vi "Untitled 1.vi"() -> ()   [LabVIEW 2015]
uses:
  <vilib>/Utility/file.llb/Read Delimited Spreadsheet (DBL).vi
panel:
  out "Multiple Plots (custom time base)":dbl[](graph)
  in  "stop":bool
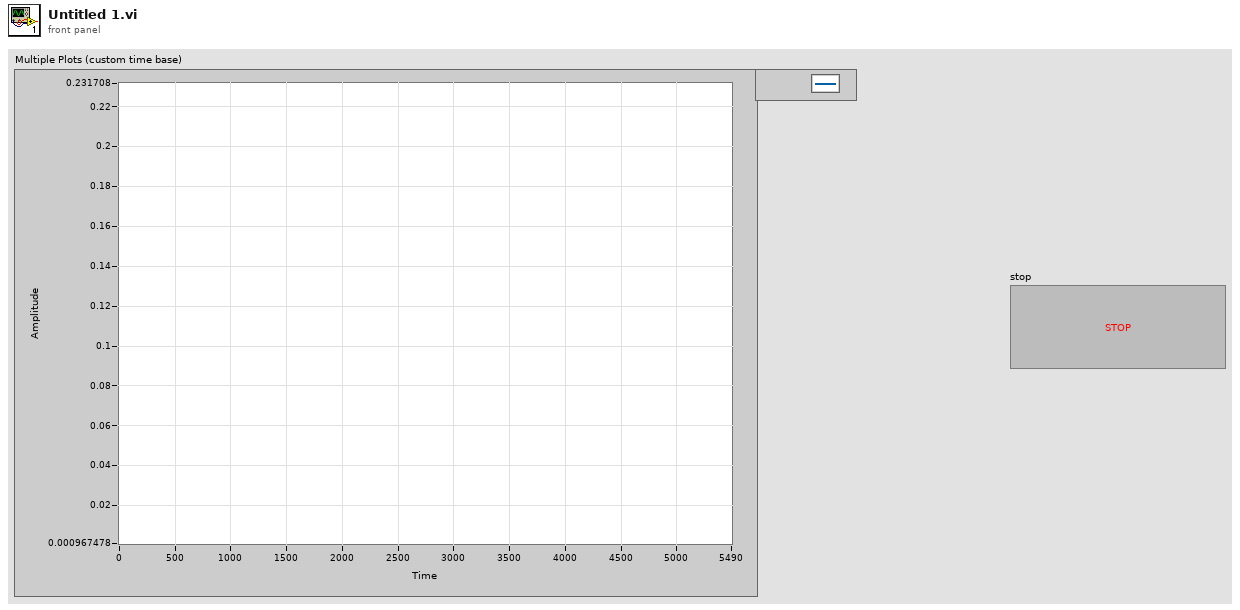
[diagram p1: front panel]
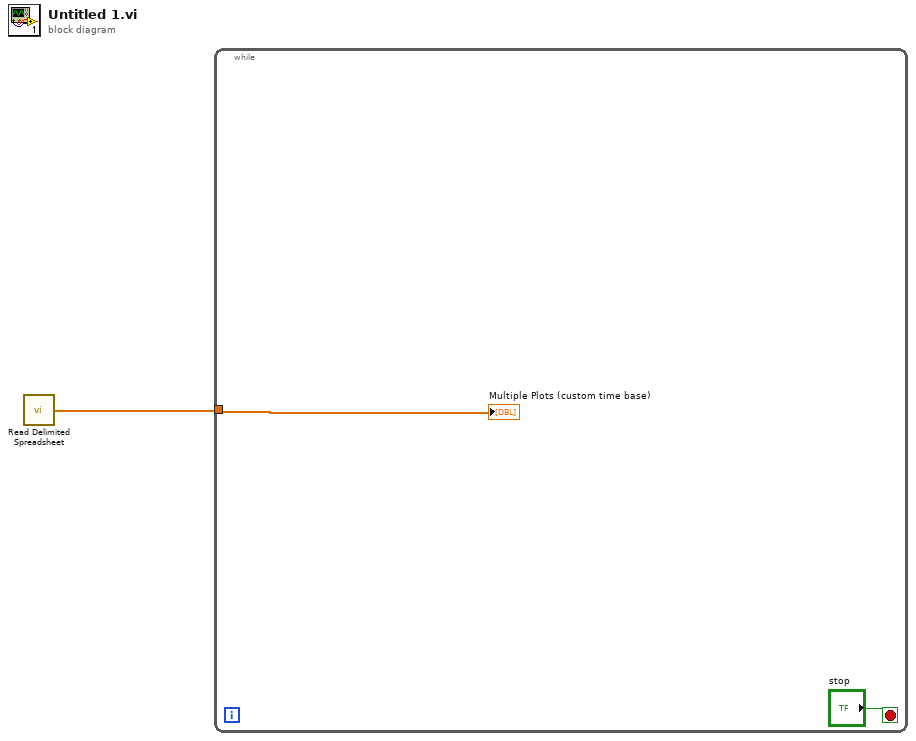
[diagram p0: block diagram]
diagram:
  n1 = call-poly <vilib>:"Read Delimited Spreadsheet.vi"() -> ("first row"=w1:dbl[])  [unwired: 10 in, 5 out]
  n2 = while {
    tunnel: w1 -> [w2]
    stop <- "stop" stop-if-true
    "Multiple Plots (custom time base)" <- w2
  }
